vi "bufferPosition.vi"(3 "Input String":string) -> (16 "Output 12":string, 17 "Output1":string, 18 "Output 11":string, 19 "Output 2":string, 20 "Output 10":string, 21 "Output 9":string, 22 "Output 8":string, 23 "Output 7":string, 24 "Output 6":string, 25 "Output 5":string, 26 "Output 4":string, 27 "Output 3":string)   [LabVIEW 2015]
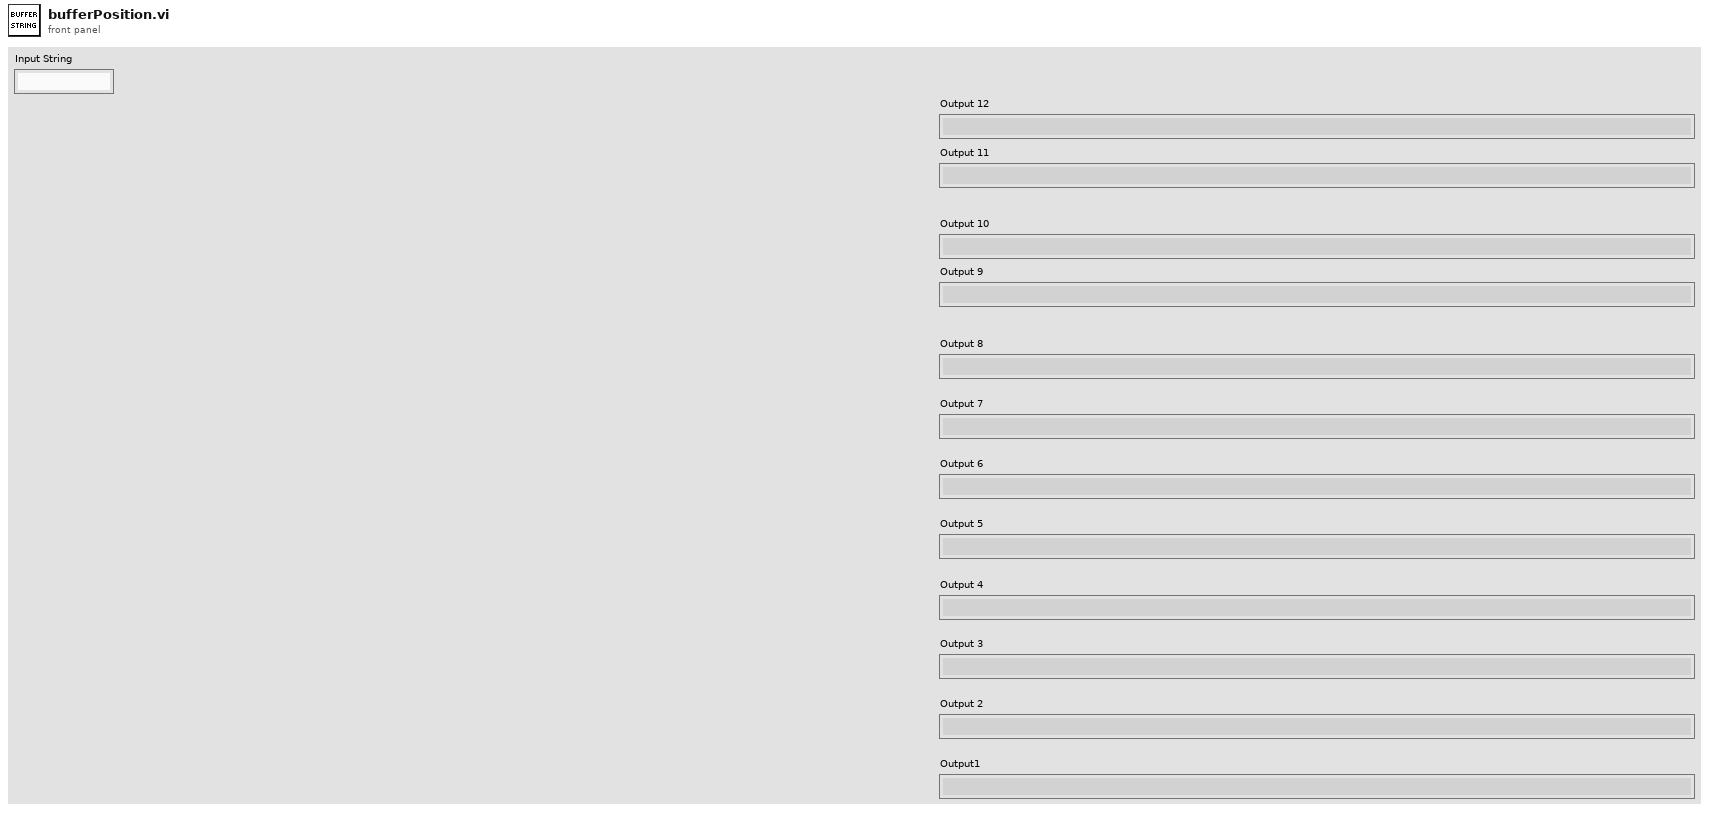
[diagram p1: front panel]
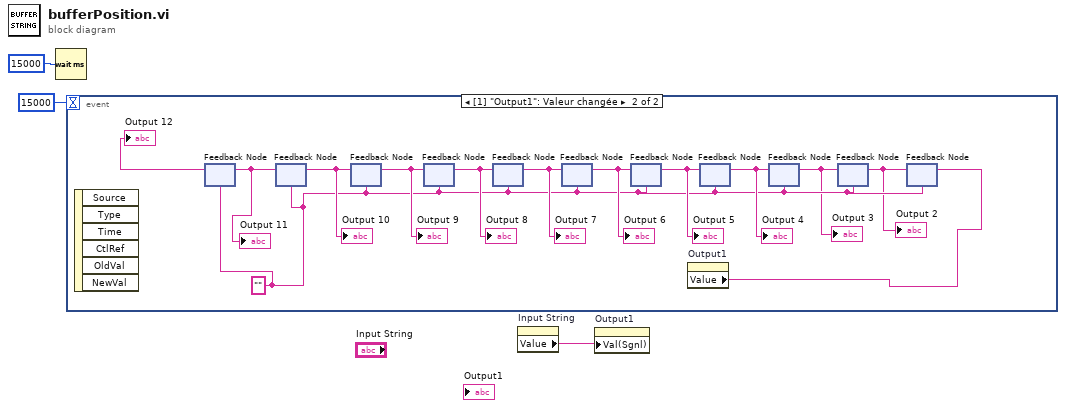
[diagram p0: block diagram]
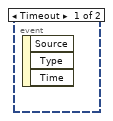
[diagram p2: hidden frame]
diagram:
  n1 = Wait (ms)(milliseconds to wait=u32 15000) -> ()  [unwired: 1 out]
  n2 = event shown="[1] \"Output1\": Valeur changée" {
    selector: _ -> [_ _]
    dyn-events: _ -> [_ _]
    timeout: 15000 -> [_ _]
    event Timeout {
      n3 = event-data() -> ()  [unwired: 1 in, 3 out]
    }
    event "Output1": Value Change {
      w9 = ""
      n4 = event-data() -> ()  [unwired: 1 in, 6 out]
      n5 = feedback #1(w9) -> (→"Output 12":string)
      n6 = feedback #2(w9) -> (w6:string)
      "Output 11" <- w6
      n7 = feedback-in #1(w6) -> ()
      n8 = feedback #3(w9) -> (w10:string)
      "Output 10" <- w10
      n9 = feedback-in #2(w10) -> ()
      n10 = feedback #4(w9) -> (w11:string)
      "Output 9" <- w11
      n11 = feedback-in #3(w11) -> ()
      n12 = feedback #5(w9) -> (w12:string)
      "Output 8" <- w12
      n13 = feedback-in #4(w12) -> ()
      n14 = feedback #6(w9) -> (w13:string)
      "Output 7" <- w13
      n15 = feedback-in #5(w13) -> ()
      n16 = feedback #7(w9) -> (w14:string)
      "Output 6" <- w14
      n17 = feedback-in #6(w14) -> ()
      n18 = property on="Output1" class="Ch"() -> ("Value"=w4:string)  [unwired: 2 in, 2 out]
      n19 = feedback #8(w9) -> (w15:string)
      "Output 5" <- w15
      n20 = feedback-in #7(w15) -> ()
      n21 = feedback #9(w9) -> (w16:string)
      "Output 4" <- w16
      n22 = feedback-in #8(w16) -> ()
      n23 = feedback #10(w9) -> (w7:string)
      "Output 3" <- w7
      n24 = feedback-in #9(w7) -> ()
      n25 = feedback #11(w9) -> (w8:string)
      "Output 2" <- w8
      n26 = feedback-in #10(w8) -> ()
      n27 = feedback-in #11(w4) -> ()
    }
  }
  n28 = property on="Input String" class="Ch"() -> ("Value"=w1:string)  [unwired: 2 in, 2 out]
  n29 = property on="Output1" class="Ch"("Val(Sgnl)"=w1) -> ()  [unwired: 2 in, 2 out]
